vi "Write All.vi"(8 "Error In":errorcluster, 10 "Data":u8[](array[numeric]), 11 "Channel In":refnum<class "Channel.lvclass">) -> (0 "Error Out":errorcluster, 2 "Write Count":u64, 3 "Channel Out":refnum<class "Channel.lvclass">)   [LabVIEW 2018, in "Toolkit.lvlib" / "Channel.lvclass"]
uses:
  Channel.lvclass
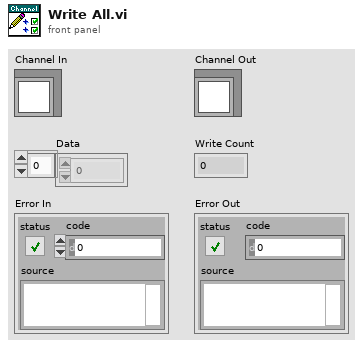
[diagram p1: front panel]
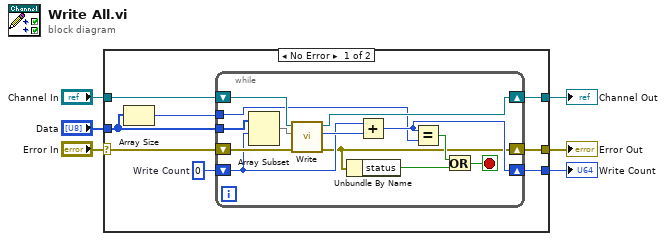
[diagram p0: block diagram]
diagram:
  n1 = case shown="No Error" "Error In" {
    selector: "Error In" -> [w8 w28]
    tunnel: "Data" -> [w12 _]
    tunnel: "Channel In" -> [w11 w29]
    tunnel: [w10 w29] -> w4
    tunnel: [w9 w28] -> w3
    tunnel: [w7 _] -> w1
    frame No Error {
      w13 = u64 0  # Write Count
      n2 = Array Size(array=w12) -> (size(s)=w14:i32)
      n3 = while {
        tunnel: w12 -> [w24]
        shift-right: [w17] -> w9
        shift-left: w8 -> [w27]
        shift-right: [w25] -> w10
        shift-left: w11 -> [w26]
        tunnel: w14 -> [w19]
        shift-right: [w20] -> w7
        shift-left: w13 -> [w21]
        stop <- w15 stop-if-true
        n4 = Array Subset(array=w24, index=w21) -> (w23:u8[])  [unwired: 1 in]
        n5 = call "Write.vi"("Error In"=w27, "Data"=w23, "Channel In"=w26) -> ("Error Out"=w17:errorcluster, "Write Count"=w22:u64, "Channel Out"=w25:refnum<class "Channel.lvclass">)  [unwired: 6 in]
        n6 = Unbundle By Name(w17) -> ("status"=w16:bool)
        n7 = Add(x=w21, y=w22) -> (x+y=w20:u64)
        n8 = Equal?(x=w20, y=w19) -> (x = y?=w18:bool)
        n9 = Or(x=w18, y=w16) -> (x .or. y?=w15:bool)
      }
    }
    frame Error {
    }
  }
  "Channel Out" <- w4
  "Error Out" <- w3
  "Write Count" <- w1
